vi "UDP Write Memory.vi"(5 "port or service name":u16, 6 "pack size(400)":i32=400, 7 "address":u32, 8 "error in (no error)":errorcluster, 9 "超时毫秒(25000)":i32=25000, 10 "String":string, 11 "UDP Network Connection in":refnum<k16>) -> (0 "error out":errorcluster, 3 "UDP Network Connection out":refnum<k16>, 4 "checksum":dbl[](array[numeric]))   [LabVIEW 2017, in "UDP++.lvlib"]
uses:
  UDP++.lvlib
  f860383b-7b7b-459c-974e-2ed9ce032f24.vi
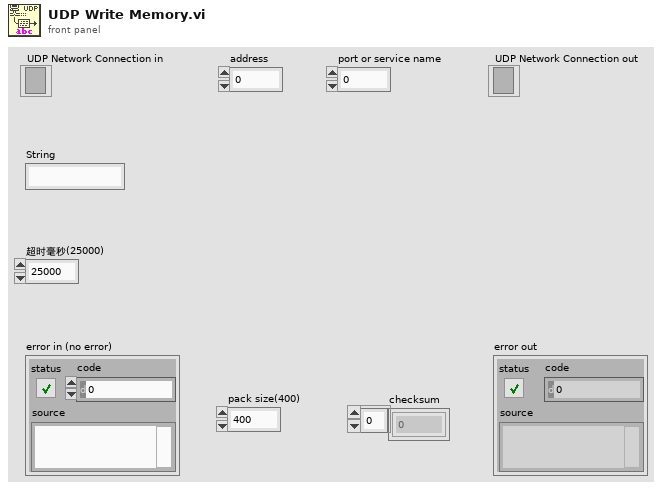
[diagram p1: front panel]
types:
  T1 = cluster{i32, i32, "String":string, "Validation":dbl}
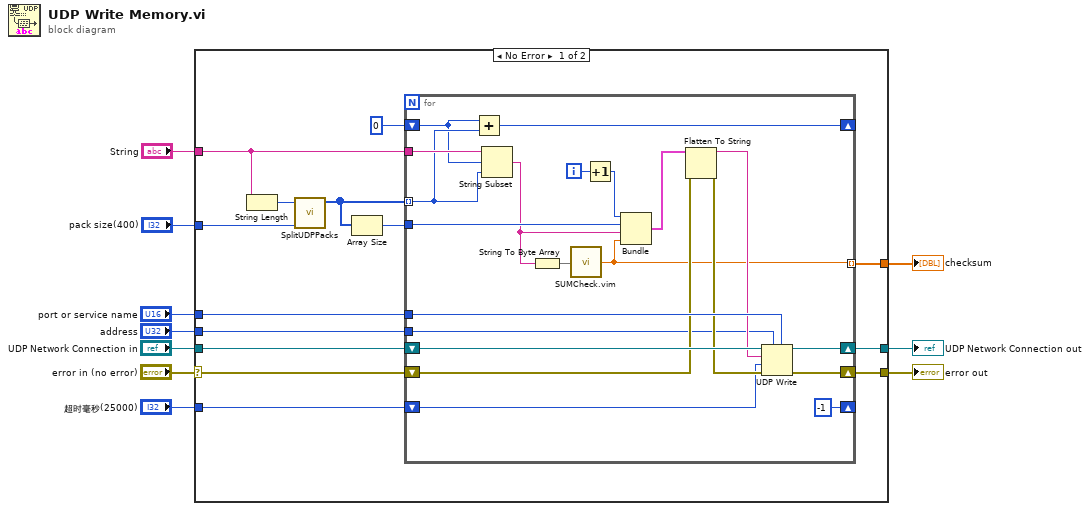
[diagram p0: block diagram]
diagram:
  n1 = case shown="No Error" "error in (no error)" {
    selector: "error in (no error)" -> [w17 w47]
    tunnel: "pack size(400)" -> [w21 _]
    tunnel: "String" -> [w20 _]
    tunnel: [w19 w47] -> w8
    tunnel: "address" -> [w18 _]
    tunnel: "port or service name" -> [w16 _]
    tunnel: [w15 w46] -> w4
    tunnel: "UDP Network Connection in" -> [w14 w46]
    tunnel: "超时毫秒(25000)" -> [w13 _]
    tunnel: [w11 _] -> w1
    frame No Error {
      n2 = String Length(string=w20) -> (length=w12:i32)
      n3 = call "SplitUDPPacks.vi"("y"=w21, "size"=w12) -> ("output array"=w22:i32[])  [unwired: 9 in]
      n4 = Array Size(array=w22) -> (size(s)=w23:i32)
      n5 = for {
        tunnel: w16 -> [w43]
        tunnel: w18 -> [w39]
        tunnel: w20 -> [w37]
        shift-right: [w44] -> w15
        shift-left: w14 -> [w45]
        shift-right: [w38] -> w19
        shift-left: w17 -> [w41]
        tunnel: w22 -> [w29] mode=indexing
        tunnel: w23 -> [w36]
        shift-right: [w33] -> _
        shift-left: 0 ("y") -> [w28]
        shift-right: [-1 ("超时毫秒(25000)")] -> _
        shift-left: w13 -> [w31]
        tunnel: [w25] -> w11 mode=indexing
        i -> [w34]
        n6 = Add(x=w28, y=w29) -> (x+y=w33:i32)
        n7 = String Subset(string=w37, offset (0)=w28, length (rest)=w29) -> (substring=w27:string)
        n8 = String To Byte Array(string=w27) -> (unsigned byte array=w26:u8[])
        n9 = call "SUMCheck.vim"("Array"=w26) -> ("Validation"=w25:dbl)
        n10 = Increment(x=w34) -> (x+1=w32:i32)
        n11 = Bundle(w32, w36, "String"=w27, "Validation"=w25) -> (w35:T1)  [unwired: 1 in]
        n12 = Flatten To String(anything=w35, error in (no error)=w41) -> (data string=w42:string, error out=w40:errorcluster)  [unwired: 2 in, 1 out]
        n13 = UDP Write(address=w39, port or service name=w43, connection ID=w45, data in=w42, 8:w40, 9:w31) -> (error out=w38:errorcluster, 3:w44:refnum<k16>)
      }
    }
    frame Error {
    }
  }
  "error out" <- w8
  "UDP Network Connection out" <- w4
  "checksum" <- w1
